vi "protocol_combined.vi"() -> ()   [LabVIEW 2016]
uses:
  dxl_x86_c.lvlib/dxl_x86_c.lvlib
panel:
  out "dynamixel2_comm_result":string
  out "dynamixel2_error":string
  out "dynamixel1_comm_result":string
  out "dynamixel1_error":string
  out "protocol_version2":dbl=2.0
  in  "value : MX (dial)\ngoal position 1":u16(knob)
  in  "ADDR_MX_\nPRESENT_POSITION":u16=36
  in  "ADDR_MX_\nGOAL_POSITION":u16=30
  in  "ADDR_MX_\nTORQUE_ENABLE":u16=24
  out "value : PRO (knob)\npresent position 2":i32(knob) scale=150000.0..-150000.0
  in  "dynamixe2_id":u8=2
  in  "device_name1":string="COM1"
  in  "ADDR_PRO_\nPRESENT_POSITION":u16=611
  in  "ADDR_PRO_\nGOAL_POSITION":u16=596
  in  "ADDR_PRO_\nTORQUE_ENABLE":u16=562
  out "protocol_version1":dbl=1.0
  out "value : MX (knob)\npresent position 1":u16(knob)
  in  "terminate":bool
  out "port_num":i32
  in  "value : PRO (dial)\ngoal position 2":i32(knob) scale=150000.0..-150000.0
  in  "dynamixel1_id":u8=1
  in  "baud_rate":i32=57600
  # "/*******************************************************************************\n* Copyright (c) 2016, ROBOTIS CO., LTD.\n* All rights reserved.\n*\n* Redistribution and use in source and binary forms, with or without\n* modification, are permitted provided that the following conditions are met:\n*\n* * Redistributions of source code must retain the above copyright notice, this\n*   list of conditions and the following disclaimer.\n*\n* * Redistributions in binary form must reproduce the above copyright notice,\n*   this list of conditions and the following disclaimer in the documentation\n*   and/or other materials provided with the distribution.\n*\n* * Neither the name of ROBOTIS nor the names of its\n*   contributors may be used to endorse or promote products derived from\n*   this software without specific prior written permission.\n*\n* THIS SOFTWARE IS PROVIDED BY THE COPYRIGHT HOLDERS AND CONTRIBUTORS \"AS IS\"\n* AND ANY EXPRESS OR IMPLIED WARRANTIES, INCLUDING, BUT NOT LIMITED TO, THE\n* IMPLIED WARRANTIES OF MERCHANTABILITY AND FITNESS FOR A PARTICULAR PURPOSE ARE\n* DISCLAIMED. IN NO EVENT SHALL THE COPYRIGHT HOLDER OR CONTRIBUTORS BE LIABLE\n* FOR ANY DIRECT, INDIRECT, INCIDENTAL, SPECIAL, EXEMPLARY, OR CONSEQUENTIAL\n* DAMAGES (INCLUDING, BUT NOT LIMITED TO, PROCUREMENT OF SUBSTITUTE GOODS OR\n* SERVICES; LOSS OF USE, DATA, OR PROFITS; OR BUSINESS INTERRUPTION) HOWEVER\n* CAUSED AND ON ANY THEORY OF LIABILITY, WHETHER IN CONTRACT, STRICT LIABILITY,\n* OR TORT (INCLUDING NEGLIGENCE OR OTHERWISE) ARISING IN ANY WAY OUT OF THE USE\n* OF THIS SOFTWARE, EVEN IF ADVISED OF THE POSSIBILITY OF SUCH DAMAGE.\n*******************************************************************************/\n\n/* Author: Ryu Woon Jung (Leon) */"
  # "Available Dynamixel model on this example : All models using Protocol 1.0 and 2.0\nThis example is designed for using a Dynamixel MX-28, a Dynamixel PRO 54-200 and an USB2DYNAMIXEL\nTo use another Dynamixel model, such as X series, see their details in E-Manual(support.robotis.com) \n   and edit \"numeric control\"s seen left with \"Edit Text\" tool.\nBe sure that properties of Dynamixel MX and PRO are already set as %% MX - ID : 1 / Baudnum : 1 (Baudrate : 1000000) , PRO - ID : 1 / Baudnum : 3 (Baudrate : 1000000)\n\nBe aware that:\nThis example configures two different control tables (especially, if it uses Dynamixel and Dynamixel PRO). It may modify critical Dynamixel parameter on the control table, if Dynamixels have wrong ID.\n\n\n1. Run example by click above \"Run\" button (below \"Edit\" menu).\n2. Drag \"dial\" then you may see the Dynamixel and \"knob\"s rotating\n3. To finish the example, press \"terminate\" button."
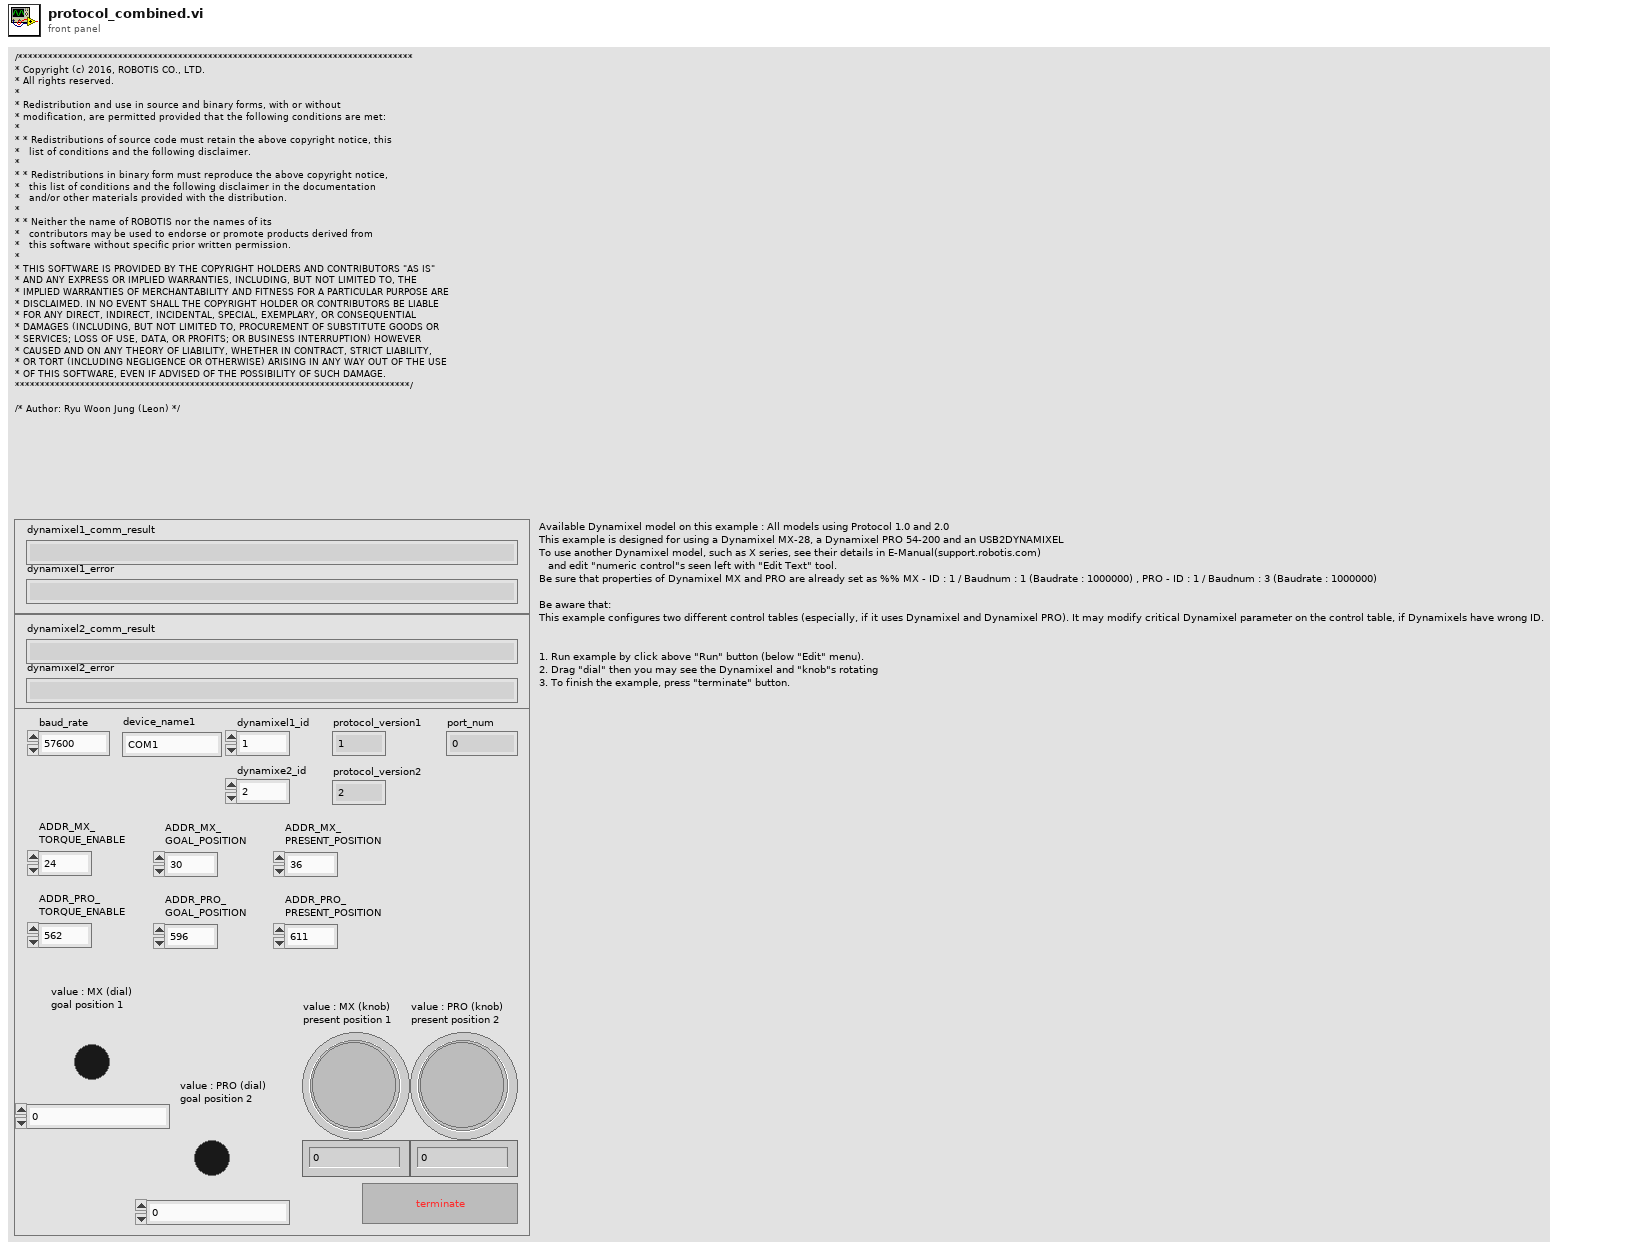
[diagram p1: front panel]
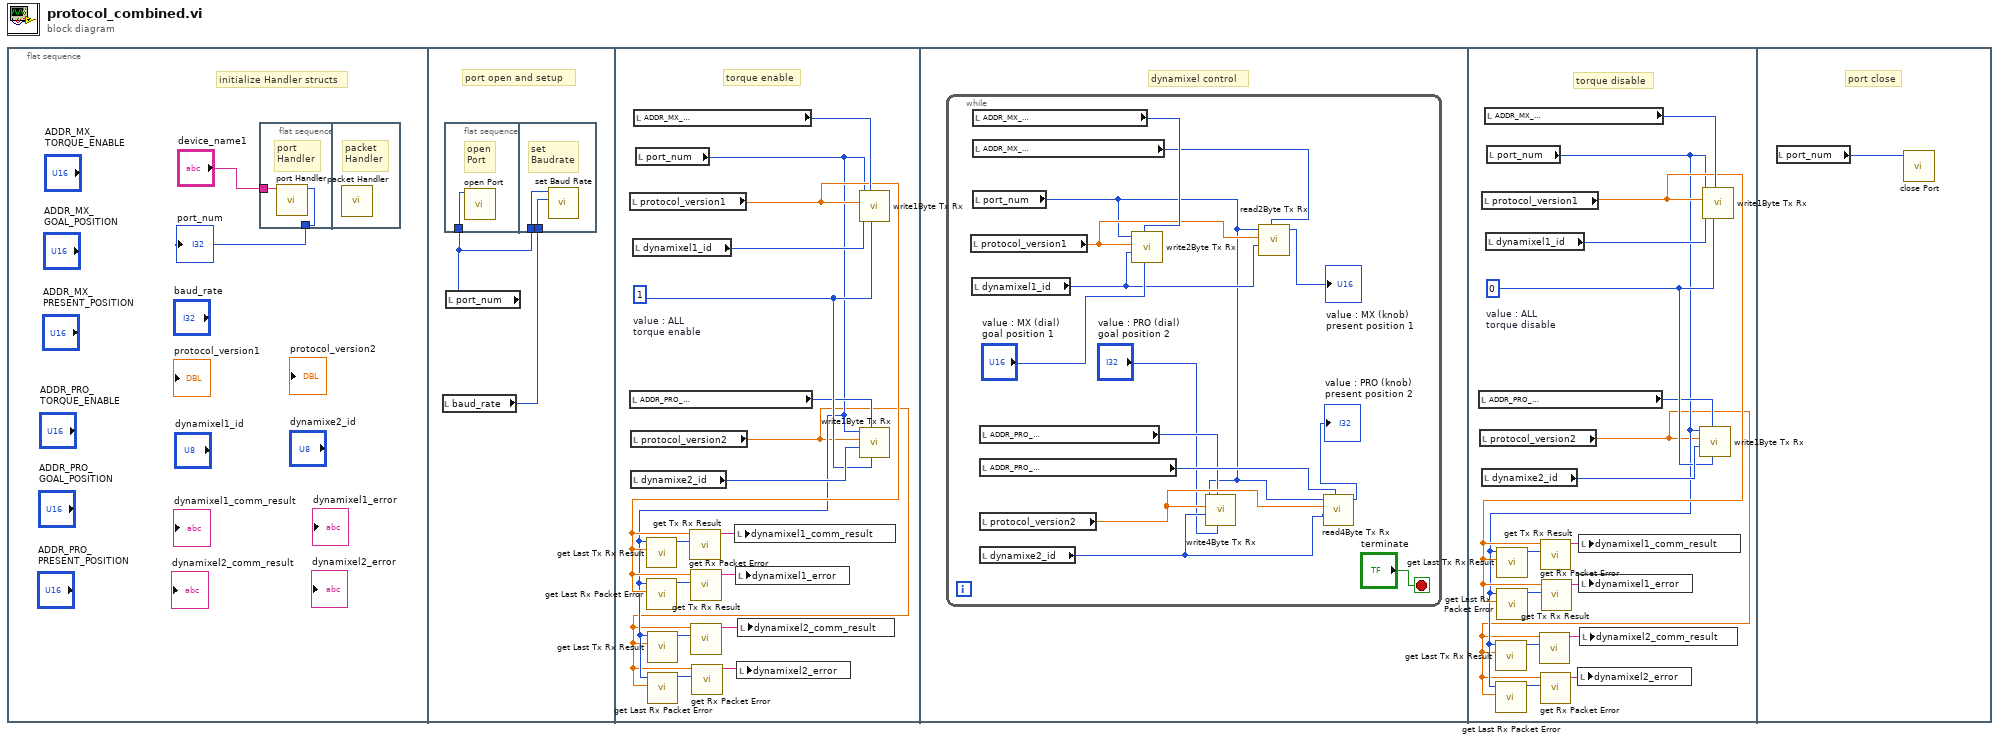
[diagram p0: block diagram]
diagram:
  n1 = flat-sequence {
    frame #0 {
      # "initialize Handler structs"
      n2 = flat-sequence {
        tunnel: "device_name1" -> [w4]
        tunnel: [w3] -> w1
        frame #0 {
          # "port\nHandler"
          n3 = call "port Handler.vi"("port_name"=w4) -> ("function return"=w3:i32)  [unwired: 10 in]
        }
        frame #1 {
          # "packet\nHandler"
          n4 = call "packet Handler.vi"() -> ()  [unwired: 12 in]
        }
      }
      "port_num" <- w1
    }
    frame #1 {
      # "port open and setup"
      n5 = local read "baud_rate"() -> (w5:i32)
      n6 = flat-sequence {
        tunnel: w6 -> [w7]
        tunnel: w6 -> [w9]
        tunnel: w5 -> [w8]
        frame #0 {
          # "open\nPort"
          n7 = call "open Port.vi"("port_num"=w7) -> ()  [unwired: 10 in, 1 out]
        }
        frame #1 {
          # "set\nBaudrate"
          n8 = call "set Baud Rate.vi"("baudrate"=w8, "port_num"=w9) -> ()  [unwired: 9 in, 1 out]
        }
      }
      n9 = local read "port_num"() -> (w6:i32)
    }
    frame #2 {
      w22 = 1  # value : ALL torque enable
      # "torque enable"
      n10 = local read "protocol_version1"() -> (w16:dbl)
      n11 = local read "ADDR_PRO_\nTORQUE_ENABLE"() -> (w21:u16)
      n12 = local read "protocol_version2"() -> (w10:dbl)
      n13 = local read "dynamixe2_id"() -> (w23:u8)
      n14 = local read "dynamixel1_id"() -> (w25:u8)
      n15 = local read "ADDR_MX_\nTORQUE_ENABLE"() -> (w24:u16)
      n16 = local read "port_num"() -> (w11:i32)
      n17 = call "get Last Tx Rx Result.vi"("protocol_version"=w16, "port_num"=w11) -> ("function return"=w17:i32)  [unwired: 9 in]
      n18 = call "get Last Rx Packet Error.vi"("protocol_version"=w16, "port_num"=w11) -> ("function return"=w18:u8)  [unwired: 9 in]
      n19 = call "get Last Tx Rx Result.vi"("protocol_version"=w10, "port_num"=w11) -> ("function return"=w12:i32)  [unwired: 9 in]
      n20 = call "get Last Rx Packet Error.vi"("protocol_version"=w10, "port_num"=w11) -> ("function return"=w13:u8)  [unwired: 9 in]
      n21 = call "get Tx Rx Result.vi"("result"=w17, "protocol_version"=w16) -> ("function return"=w19:string)  [unwired: 9 in]
      n22 = call "get Rx Packet Error.vi"("error"=w18, "protocol_version"=w16) -> ("function return"=w20:string)  [unwired: 9 in]
      n23 = call "get Tx Rx Result.vi"("result"=w12, "protocol_version"=w10) -> ("function return"=w14:string)  [unwired: 9 in]
      n24 = call "get Rx Packet Error.vi"("error"=w13, "protocol_version"=w10) -> ("function return"=w15:string)  [unwired: 9 in]
      n25 = local write "dynamixel1_comm_result"(w19) -> ()
      n26 = local write "dynamixel1_error"(w20) -> ()
      n27 = local write "dynamixel2_error"(w15) -> ()
      n28 = local write "dynamixel2_comm_result"(w14) -> ()
      n29 = call "write1Byte Tx Rx.vi"("data"=w22, "address"=w24, "id"=w25, "protocol_version"=w16, "port_num"=w11) -> ()  [unwired: 7 in]
      n30 = call "write1Byte Tx Rx.vi"("data"=w22, "address"=w21, "id"=w23, "protocol_version"=w10, "port_num"=w11) -> ()  [unwired: 7 in]
    }
    frame #3 {
      # "dynamixel control"
      n31 = while {
        stop <- "terminate" stop-if-true
        n32 = local read "protocol_version1"() -> (w28:dbl)
        n33 = local read "dynamixel1_id"() -> (w27:u8)
        n34 = local read "ADDR_MX_\nGOAL_POSITION"() -> (w36:u16)
        n35 = local read "ADDR_MX_\nPRESENT_POSITION"() -> (w30:u16)
        n36 = local read "port_num"() -> (w26:i32)
        n37 = local read "ADDR_PRO_\nGOAL_POSITION"() -> (w33:u16)
        n38 = local read "ADDR_PRO_\nPRESENT_POSITION"() -> (w34:u16)
        n39 = local read "protocol_version2"() -> (w35:dbl)
        n40 = local read "dynamixe2_id"() -> (w37:u8)
        n41 = call "write2Byte Tx Rx.vi"("data"="value : MX (dial)\ngoal position 1", "address"=w36, "id"=w27, "protocol_version"=w28, "port_num"=w26) -> ()  [unwired: 7 in]
        n42 = call "write4Byte Tx Rx.vi"("data"="value : PRO (dial)\ngoal position 2", "address"=w33, "id"=w37, "protocol_version"=w35, "port_num"=w26) -> ()  [unwired: 7 in]
        n43 = call "read2Byte Tx Rx.vi"("address"=w30, "id"=w27, "protocol_version"=w28, "port_num"=w26) -> ("function return"=→"value : MX (knob)\npresent position 1":u16)  [unwired: 7 in]
        n44 = call "read4Byte Tx Rx.vi"("address"=w34, "id"=w37, "protocol_version"=w35, "port_num"=w26) -> ("function return"=→"value : PRO (knob)\npresent position 2":u32)  [unwired: 7 in]
      }
    }
    frame #4 {
      w52 = 0  # value : ALL torque disable
      # "torque disable"
      n45 = local read "ADDR_PRO_\nTORQUE_ENABLE"() -> (w51:u16)
      n46 = local read "protocol_version2"() -> (w40:dbl)
      n47 = local read "protocol_version1"() -> (w46:dbl)
      n48 = local read "dynamixe2_id"() -> (w53:u8)
      n49 = local read "ADDR_MX_\nTORQUE_ENABLE"() -> (w54:u16)
      n50 = local read "dynamixel1_id"() -> (w55:u8)
      n51 = local read "port_num"() -> (w41:i32)
      n52 = call "get Last Tx Rx Result.vi"("protocol_version"=w40, "port_num"=w41) -> ("function return"=w43:i32)  [unwired: 9 in]
      n53 = call "get Last Rx Packet Error.vi"("protocol_version"=w40, "port_num"=w41) -> ("function return"=w42:u8)  [unwired: 9 in]
      n54 = call "get Last Tx Rx Result.vi"("protocol_version"=w46, "port_num"=w41) -> ("function return"=w48:i32)  [unwired: 9 in]
      n55 = call "get Last Rx Packet Error.vi"("protocol_version"=w46, "port_num"=w41) -> ("function return"=w47:u8)  [unwired: 9 in]
      n56 = call "get Tx Rx Result.vi"("result"=w43, "protocol_version"=w40) -> ("function return"=w44:string)  [unwired: 9 in]
      n57 = call "get Tx Rx Result.vi"("result"=w48, "protocol_version"=w46) -> ("function return"=w49:string)  [unwired: 9 in]
      n58 = call "get Rx Packet Error.vi"("error"=w42, "protocol_version"=w40) -> ("function return"=w45:string)  [unwired: 9 in]
      n59 = call "get Rx Packet Error.vi"("error"=w47, "protocol_version"=w46) -> ("function return"=w50:string)  [unwired: 9 in]
      n60 = local write "dynamixel2_error"(w45) -> ()
      n61 = local write "dynamixel1_comm_result"(w49) -> ()
      n62 = local write "dynamixel1_error"(w50) -> ()
      n63 = local write "dynamixel2_comm_result"(w44) -> ()
      n64 = call "write1Byte Tx Rx.vi"("data"=w52, "address"=w51, "id"=w53, "protocol_version"=w40, "port_num"=w41) -> ()  [unwired: 7 in]
      n65 = call "write1Byte Tx Rx.vi"("data"=w52, "address"=w54, "id"=w55, "protocol_version"=w46, "port_num"=w41) -> ()  [unwired: 7 in]
    }
    frame #5 {
      # "port close"
      n66 = local read "port_num"() -> (w56:i32)
      n67 = call "close Port.vi"("port_num"=w56) -> ()  [unwired: 11 in]
    }
  }
